vi "BTS 2.vi"() -> ()   [LabVIEW 2024]
panel:
  in  "Numeric 3":dbl
  in  "stop 2":bool
  out "Numeric 2":i32
  in  "delay 2":u32
  in  "°F 2":dbl(slide) scale=0.0..300.0
  out "°C 2":dbl(slide) scale=-100.0..150.0
  in  "Boolean":bool
  out "°C":dbl(slide) scale=-100.0..150.0
  in  "°F":dbl(slide) scale=0.0..300.0
  in  "delay":u32
  out "Numeric":i32
  in  "stop":bool
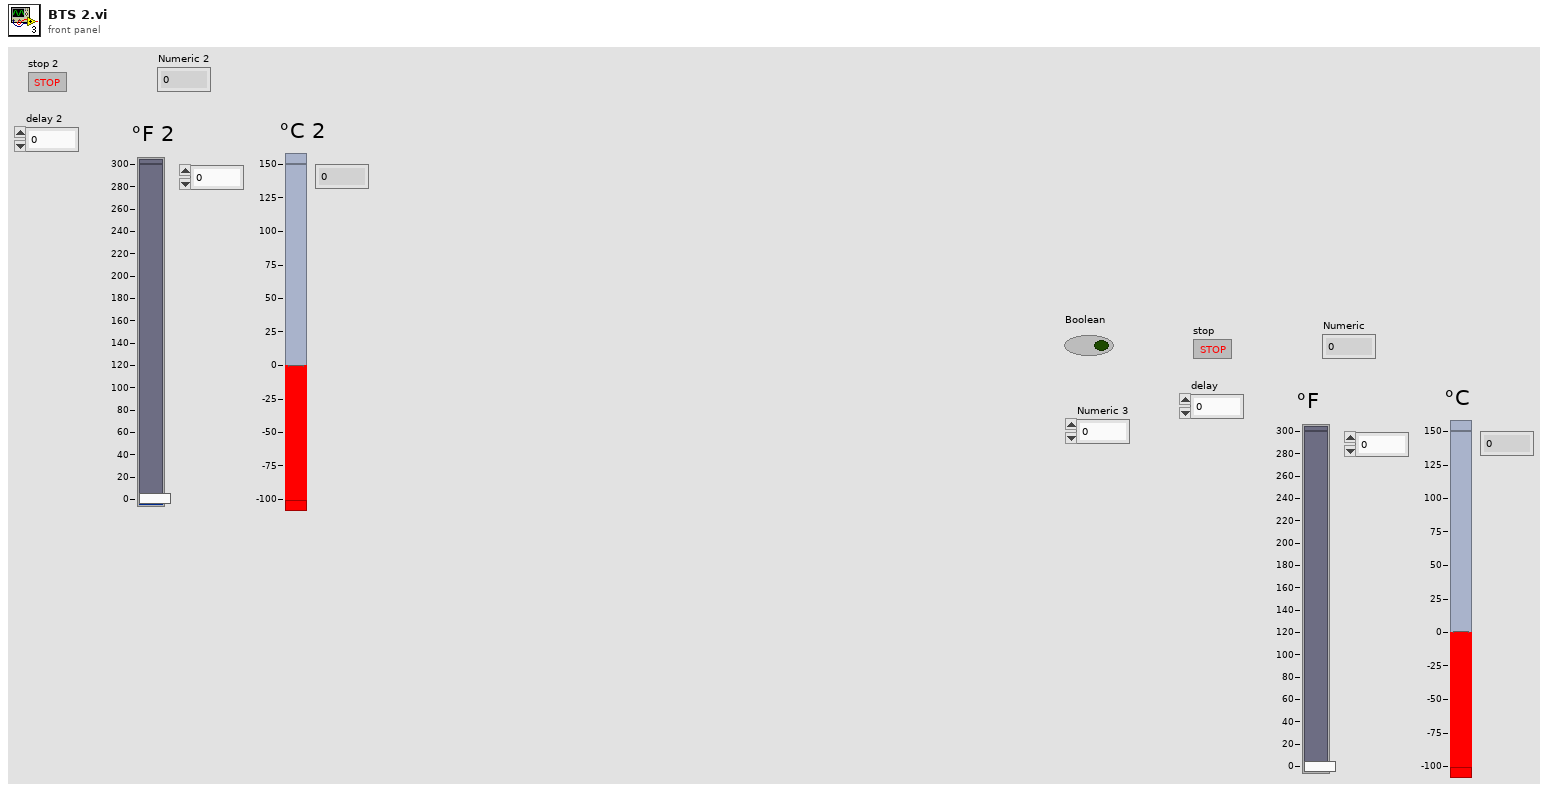
[diagram p1: front panel]
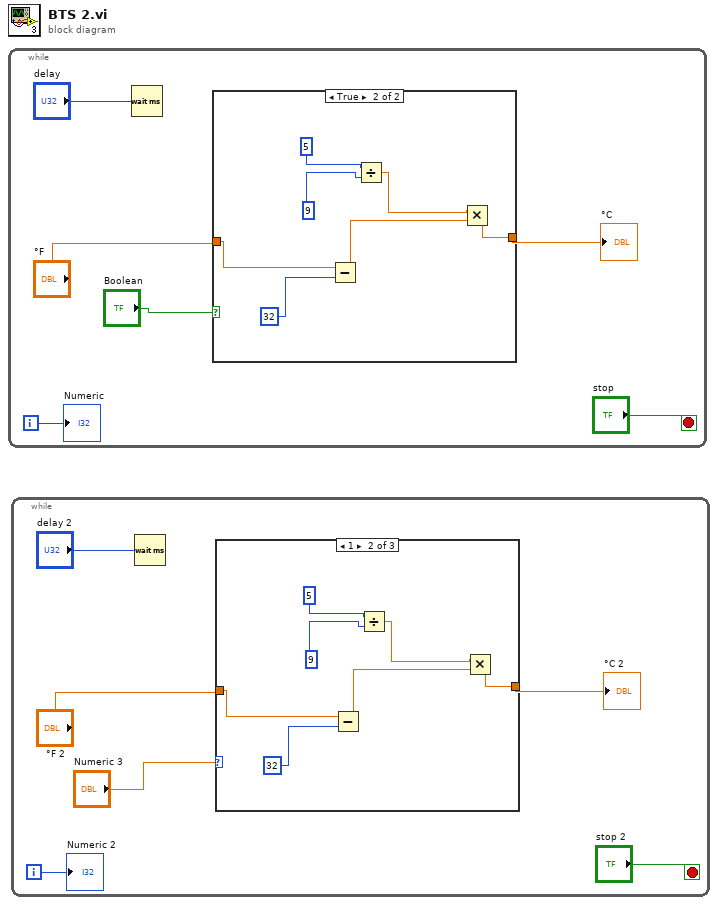
[diagram p0: block diagram]
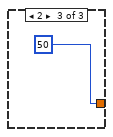
[diagram p3: hidden frame]
diagram:
  n1 = while {
    i -> [w5]
    stop <- "stop" stop-if-true
    n2 = Wait (ms)(milliseconds to wait="delay") -> ()  [unwired: 1 out]
    n3 = case shown="True" "Boolean" {
      tunnel: "°F" -> [w7 w14]
      tunnel: [w7 w8] -> w2
      frame False {
      }
      frame True {
        n4 = Subtract(x=w14, y=32) -> (x-y=w9:dbl)
        n5 = Divide(x=5, y=9) -> (x/y=w10:dbl)
        n6 = Multiply(x=w10, y=w9) -> (x*y=w8:dbl)
      }
    }
    "°C" <- w2
    "Numeric" <- w5
  }
  n7 = while {
    i -> [w19]
    stop <- "stop 2" stop-if-true
    n8 = Wait (ms)(milliseconds to wait="delay 2") -> ()  [unwired: 1 out]
    n9 = case shown="1" "Numeric 3" {
      tunnel: "°F 2" -> [w21 w28 _]
      tunnel: [w21 w22 50] -> w16
      frame 0, Default {
      }
      frame 1 {
        n10 = Subtract(x=w28, y=32) -> (x-y=w23:dbl)
        n11 = Divide(x=5, y=9) -> (x/y=w24:dbl)
        n12 = Multiply(x=w24, y=w23) -> (x*y=w22:dbl)
      }
      frame 2 {
      }
    }
    "°C 2" <- w16
    "Numeric 2" <- w19
  }
